vi "FTW-ERR-SerializeForLog.vi"(1 "error in":errorcluster) -> (0 "Serialized Error":string)   [LabVIEW 2014]
panel:
  # "Inputs"
  # "Outputs"
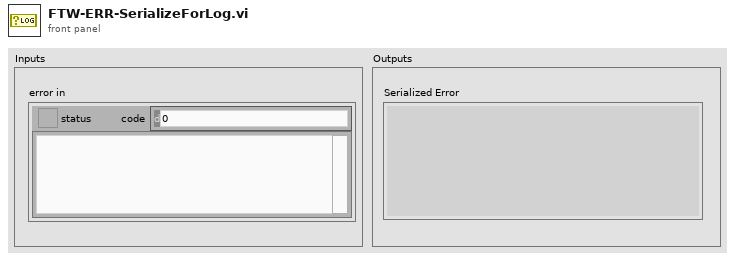
[diagram p1: front panel]
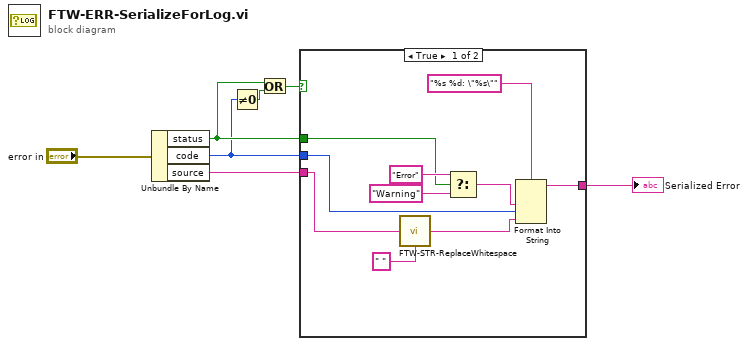
[diagram p0: block diagram]
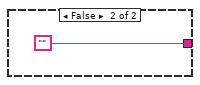
[diagram p2: hidden frame]
diagram:
  n1 = Unbundle By Name("error in") -> ("status"=w3:bool, "code"=w2:i32, "source"=w1:string)
  n2 = Not Equal To 0?(x=w2) -> (x != 0?=w4:bool)
  n3 = Or(x=w3, y=w4) -> (x .or. y?=w6:bool)
  n4 = case shown="True" w6 {
    tunnel: [w15 ""] -> w7
    tunnel: w3 -> [w9 _]
    tunnel: w2 -> [w13 _]
    tunnel: w1 -> [w14 _]
    frame True {
      n5 = call "FTW-STR-ReplaceWhitespace.vi"("Replace Spaces With..."=" ", "Input"=w14) -> ("Output"=w17:string)  [unwired: 2 in]
      n6 = Select(t="Error", s=w9, f="Warning") -> (s? t:f=w10:string)
      n7 = Format Into String(format string="%s %d: \"%s\"", w10, w13, w17) -> (resulting string=w15:string)  [unwired: 2 in, 1 out]
    }
    frame False {
    }
  }
  "Serialized Error" <- w7
